vi "AdditionCode.vi"() -> ()   [LabVIEW 2020]
panel:
  out "y 2":dbl(knob) scale=0.0..10.0
  out "Waveform Chart":dbl(graph)
  in  "y":dbl(slide) scale=0.0..10.0
  in  "x":dbl
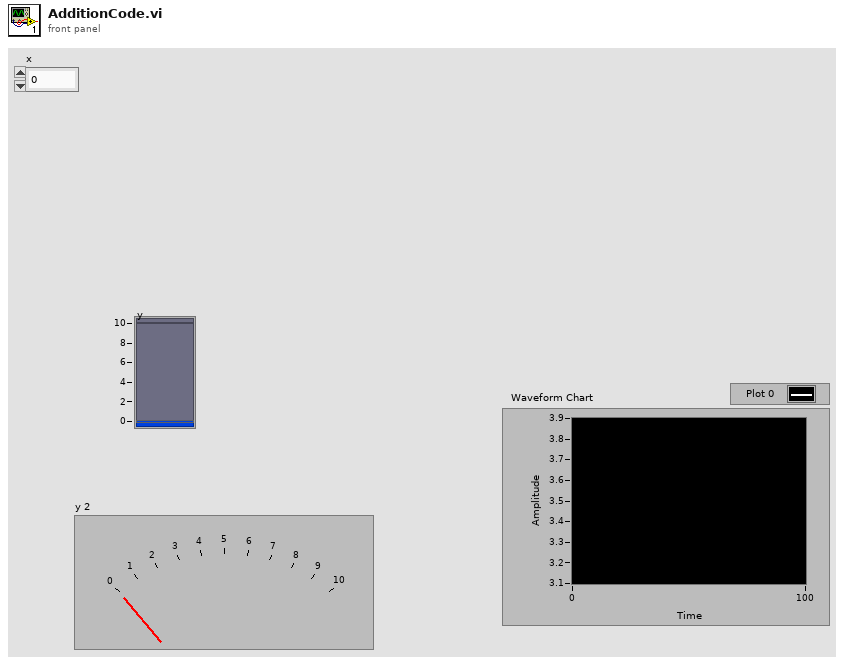
[diagram p1: front panel]
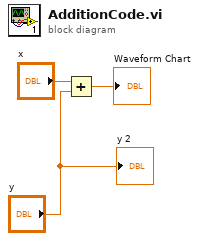
[diagram p0: block diagram]
diagram:
  n1 = Add(x="x", y="y") -> (x+y=→"Waveform Chart":dbl)
  "y 2" <- "y"
